vi "Lab.06_EMG.vi"() -> ()   [LabVIEW 2016]
uses:
  <vilib>/Analysis/2dsp.llb/Power Spectrum (DBL).vi
  <vilib>/measure/maspectr.llb/FFT Power Spectrum and PSD for N Chan.vi
  <vilib>/measure/NI_MAPro.lvlib
  <vilib>/Analysis/NI_AALPro.lvlib
panel:
  out "Numeric":dbl
  out "amplitude":dbl
  out "Boolean":bool
  out "Waveform Graph 2":cluster{"f0":dbl, "df":dbl, "magnitude":dbl[]}[](graph)
  out "Waveform Graph":dbl[](graph)
  in  "stop":bool
  out "Waveform Chart":dynamicdata(graph)
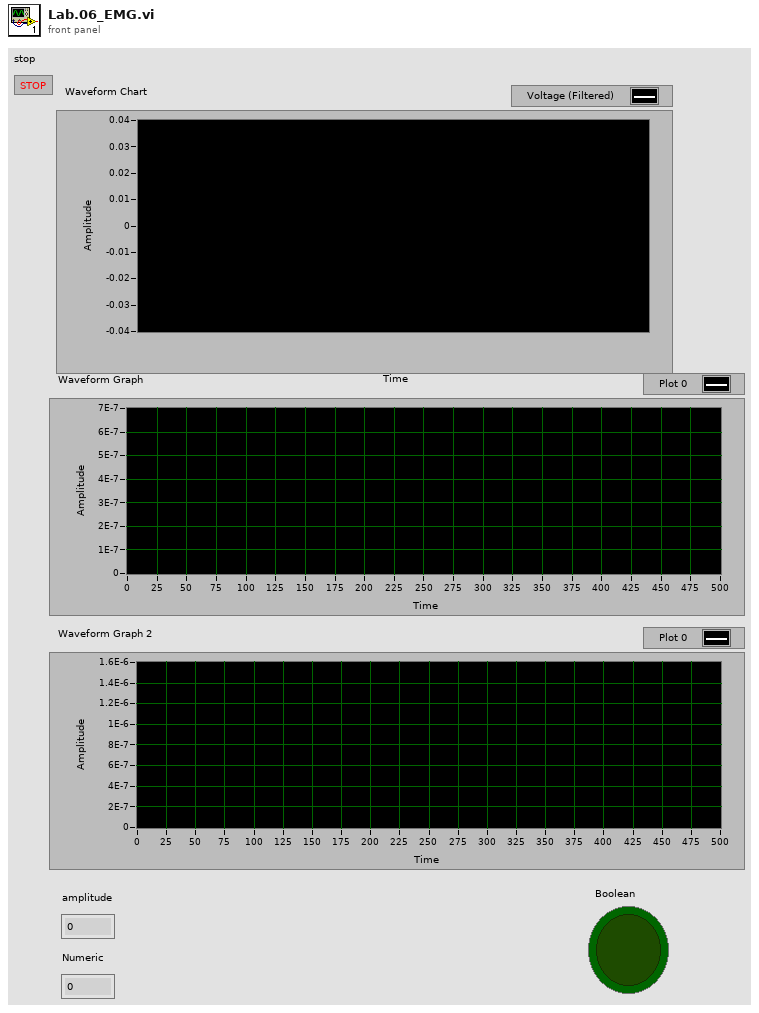
[diagram p1: front panel]
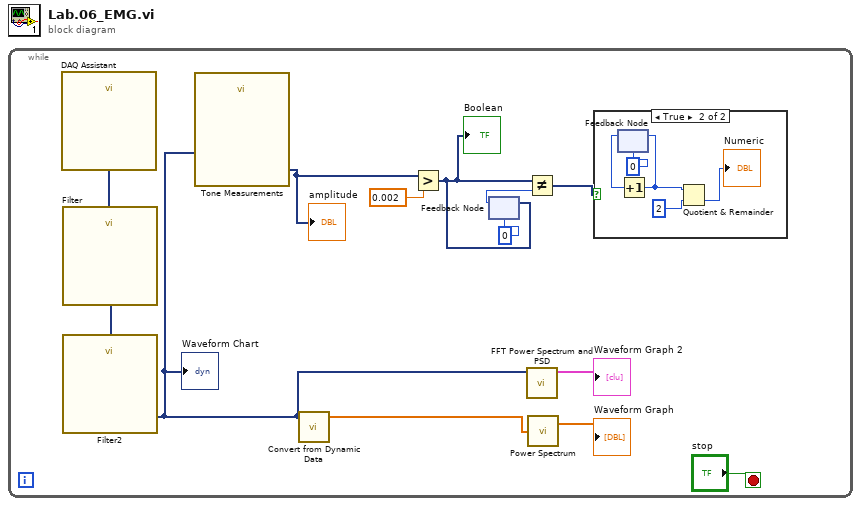
[diagram p0: block diagram]
diagram:
  n1 = while {
    stop <- "stop" stop-if-true
    n2 = call "DAQ Assistant"() -> ("data"=w13:dynamicdata)  [unwired: 16 in, 3 out]
    n3 = call "Filter"("Signal"=w13) -> ("Filtered Signal"=w11:dynamicdata)  [unwired: 9 in, 1 out]
    n4 = call "Filter2"("Signal"=w11) -> ("Filtered Signal"=w6:dynamicdata)  [unwired: 9 in, 1 out]
    "Waveform Chart" <- w6
    n5 = call "Tone Measurements"("Signals"=w6) -> ("Amplitude"=w5:dynamicdata)  [unwired: 9 in, 1 out]
    "amplitude" <- w5
    n6 = call "Convert from Dynamic Data"("Dynamic Data Type"=w6) -> ("Array"=w9:dbl[])  [unwired: 3 in]
    n7 = Greater?(x=w5, y=0.002) -> (0:w4:dynamicdata)
    "Boolean" <- w4
    n8 = feedback-in #1(w4) -> ()
    n9 = feedback #1(0) -> (w3:i32)
    n10 = Not Equal?(x=w4, y=w3) -> (x != y?=w2:dynamicdata)
    n11 = call-poly <vilib>:"FFT Power Spectrum and PSD.vi"("time signals"=w6) -> ("Power Spectrum / PSD"=→"Waveform Graph 2":cluster{"f0":dbl, "df":dbl, "magnitude":dbl[]}[])  [unwired: 7 in, 3 out]
    n12 = call-poly <vilib>:"Power Spectrum.vi"("X"=w9) -> ("Power Spectrum"=→"Waveform Graph":dbl[])  [unwired: 1 out]
    n13 = case shown="True" w2 {
      frame False {
      }
      frame True {
        n14 = feedback #2(0) -> (w18:i32)
        n15 = Increment(x=w18) -> (x+1=w16:i32)
        n16 = feedback-in #2(w16) -> ()
        n17 = Quotient & Remainder(x=w16, y=2) -> (floor(x/y)=→"Numeric":i32)  [unwired: 1 out]
      }
    }
  }
